vi "evaluateParseXML.vi"(8 "error in":errorcluster, 9 "Default VData":variant, 10 "XML string":string, 11 "reference in":refnum<class "EasyXML_XML_Subset_Evaluations.lvclass">) -> (0 "error out":errorcluster, 1 "LabVIEW Data":variant, 3 "reference out":refnum<class "EasyXML_XML_Subset_Evaluations.lvclass">)   [LabVIEW 2013, in "EasyXML_XML_Subset_Evaluations.lvclass"]
uses:
  EasyXML_XML_Subset_Evaluations.lvclass
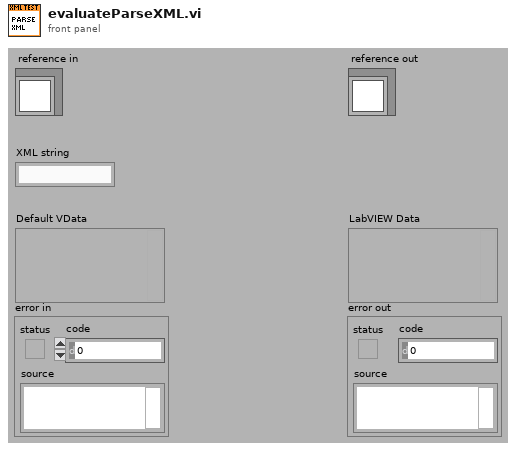
[diagram p1: front panel]
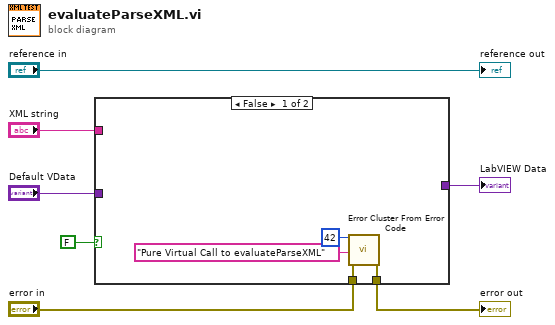
[diagram p0: block diagram]
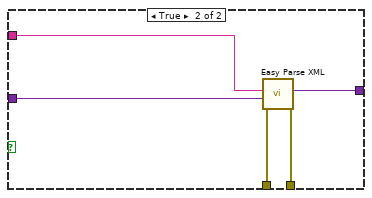
[diagram p2: hidden frame]
diagram:
  n1 = case shown="False" FALSE {
    tunnel: [_ w16] -> w6
    tunnel: "XML string" -> [_ w15]
    tunnel: [w11 w14] -> w4
    tunnel: "Default VData" -> [_ w13]
    tunnel: "error in" -> [w10 w12]
    frame False {
      n2 = call <vilib>:"Error Cluster From Error Code.vi"("error in (no error)"=w10, "error message (\"\")"="Pure Virtual Call to evaluateParseXML" ("error message (\"\")"), "error code (0)"=42) -> ("error out"=w11:errorcluster)  [unwired: 6 in]
    }
    frame True {
      n3 = call "Easy Parse XML.vi"("error in (no error)"=w12, "LabVIEW Data (Type)"=w13, "XML String"=w15) -> ("error out"=w14:errorcluster, "LabVIEW Data"=w16:variant)  [unwired: 7 in]
    }
  }
  "LabVIEW Data" <- w6
  "error out" <- w4
  "reference out" <- "reference in"
